vi "ex1.vi"() -> ()   [LabVIEW 2019]
panel:
  out "Array":bool[](array[boolean])
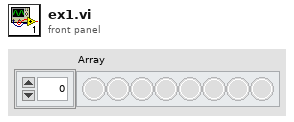
[diagram p1: front panel]
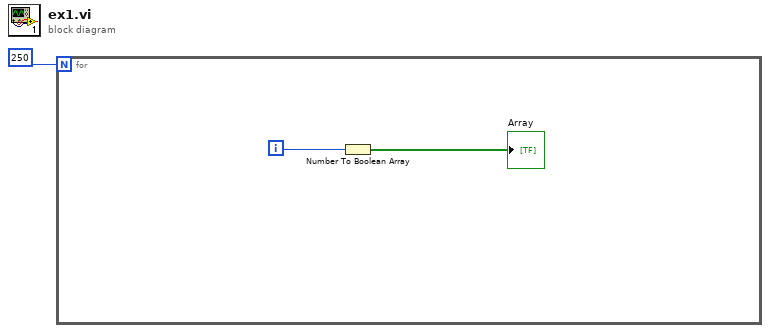
[diagram p0: block diagram]
diagram:
  n1 = for {
    N: 250 -> [_]
    i -> [w2]
    n2 = Number To Boolean Array(number=w2) -> (Boolean array=→"Array":bool[])
  }
